vi "02_get_load_save.vi"() -> ()   [LabVIEW 2025]
uses:
  d34d51db-824d-4699-8c31-a07e0fcb91a3.vi
panel:
  out "NOTIFY_UI_Main_Switch_Buttons":T1
  out "var_New_Data":bool
types:
  T1 = cluster{"button_serial_connect":bool, "button_auto_sweep":bool, "button_tcp_connect":bool}
  T2 = cluster{"button_load_sxp":bool, "button_load_csv":bool, "button_save_s1p":bool, "button_save_s2p":bool, "button_single_sweep":bool, "tcp_load_cal":bool}
  T3 = cluster{"s11_data_available":bool, "s21_data_available":bool}
  T4 = cluster{"s11_available":bool, "s21_available":bool}
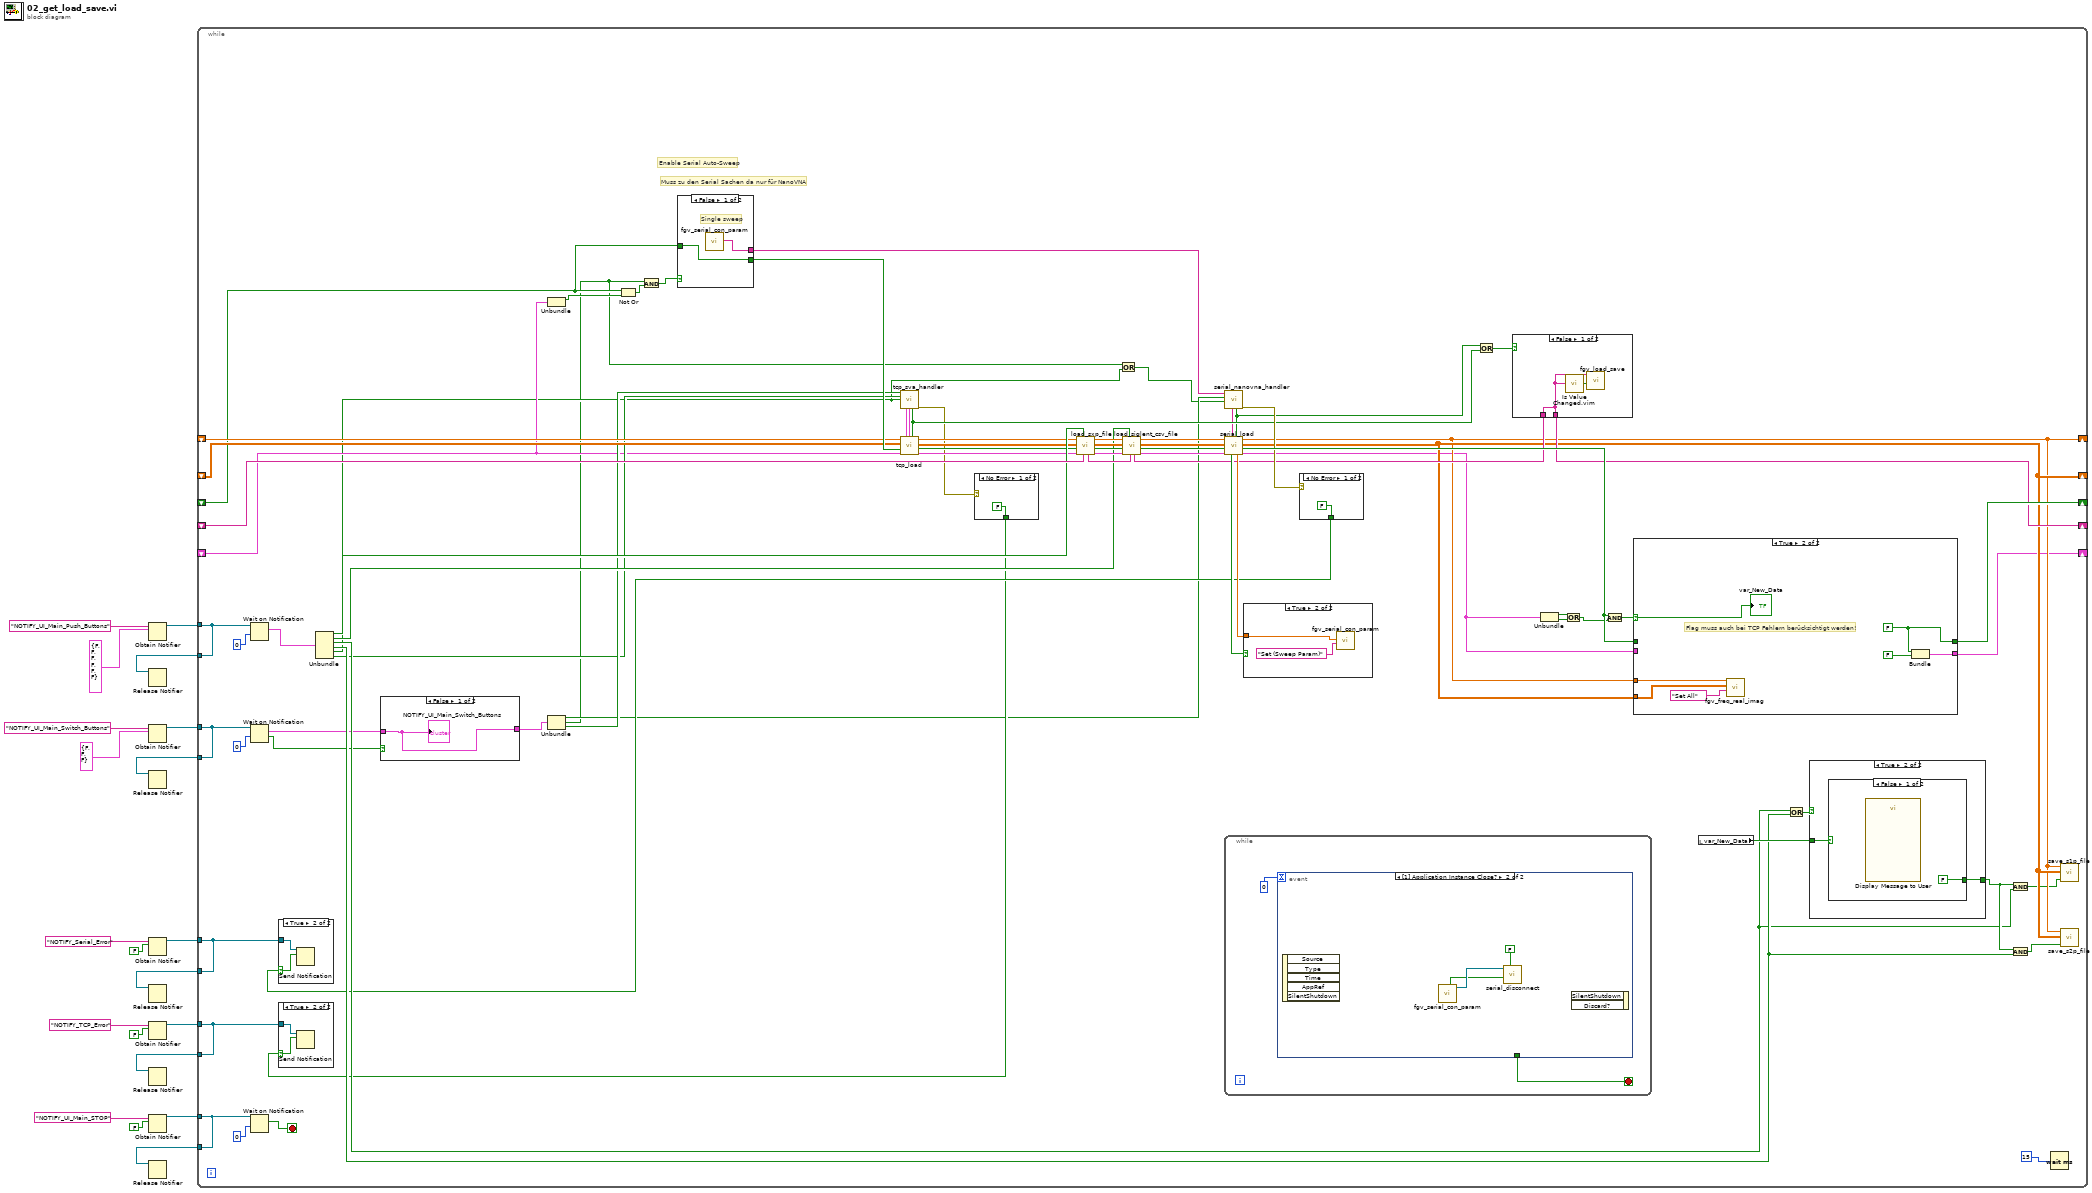
[diagram p0: block diagram]
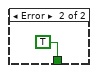
[diagram p2: hidden frame]
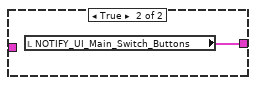
[diagram p4: hidden frame]
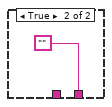
[diagram p6: hidden frame]
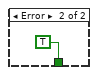
[diagram p7: hidden frame]
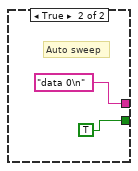
[diagram p8: hidden frame]
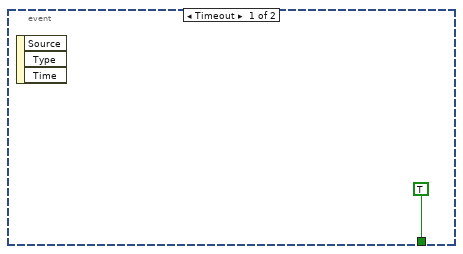
[diagram p10: hidden frame]
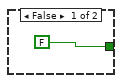
[diagram p11: hidden frame]
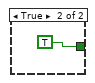
[diagram p12: hidden frame]
diagram:
  n1 = Obtain Notifier(name (unnamed)="NOTIFY_UI_Main_Push_Buttons", notification data type=T2 {"button_load_sxp"=FALSE, "button_load_csv"=FALSE, "button_save_s1p"=FALSE, "button_save_s2p"=FALSE, "button_single_sweep"=FALSE, "tcp_load_cal"=FALSE} ("output cluster")) -> (notifier out=w18:refnum<notifier>)  [unwired: 2 in, 2 out]
  n2 = Obtain Notifier(name (unnamed)="NOTIFY_UI_Main_Switch_Buttons", notification data type=T1 {"button_serial_connect"=FALSE, "button_auto_sweep"=FALSE, "button_tcp_connect"=FALSE} ("output cluster")) -> (notifier out=w9:refnum<notifier>)  [unwired: 2 in, 2 out]
  n3 = Obtain Notifier(name (unnamed)="NOTIFY_Serial_Error", notification data type=FALSE) -> (notifier out=w13:refnum<notifier>)  [unwired: 2 in, 2 out]
  n4 = Obtain Notifier(name (unnamed)="NOTIFY_TCP_Error", notification data type=FALSE) -> (notifier out=w1:refnum<notifier>)  [unwired: 2 in, 2 out]
  n5 = Obtain Notifier(name (unnamed)="NOTIFY_UI_Main_STOP", notification data type=FALSE) -> (notifier out=w14:refnum<notifier>)  [unwired: 2 in, 2 out]
  n6 = while {
    shift-right: [w95] -> _
    shift-left: _ -> [w24]
    shift-right: [w69] -> _
    shift-left: _ -> [w72]
    shift-right: [w70] -> _
    shift-left: _ -> [w73]
    shift-right: [w75] -> _
    shift-left: _ -> [w78]
    shift-right: [w63] -> _
    shift-left: _ -> [w28]
    tunnel: w18 -> [w57]
    tunnel: [w57] -> w19
    tunnel: w14 -> [w55]
    tunnel: [w55] -> w17
    tunnel: w13 -> [w48]
    tunnel: [w48] -> w10
    tunnel: w9 -> [w46]
    tunnel: [w46] -> w8
    tunnel: w1 -> [w37]
    tunnel: [w37] -> w4
    stop <- w53 stop-if-true
    # "Muss zu den Serial Sachen da nur für NanoVNA"
    # "Enable Serial Auto-Sweep"
    n7 = Wait on Notification(notifier=w57, timeout in ms (-1)=0) -> (notification=w56:T2)  [unwired: 2 in, 3 out]
    n8 = Wait on Notification(notifier=w46, timeout in ms (-1)=0) -> (notification=w43:T1, timed out?=w44:bool)  [unwired: 2 in, 2 out]
    n9 = Wait on Notification(notifier=w55, timeout in ms (-1)=0) -> (notification=w53:bool)  [unwired: 2 in, 3 out]
    n10 = Unbundle(w56) -> ("button_load_sxp"=w52:bool, "button_load_csv"=w51:bool, "button_save_s1p"=w49:bool, "button_save_s2p"=w50:bool, "button_single_sweep"=w23:bool, "tcp_load_cal"=w29:bool)
    n11 = case shown="False" w44 {
      tunnel: w43 -> [w101 _]
      tunnel: [w101 w102] -> w42
      frame False {
        "NOTIFY_UI_Main_Switch_Buttons" <- w101
      }
      frame True {
        n12 = local read "NOTIFY_UI_Main_Switch_Buttons"() -> (w102:T1)
      }
    }
    n13 = Unbundle(w28) -> ("s11_available"=w30:bool)  [unwired: 1 out]
    n14 = Unbundle(w42) -> ("button_serial_connect"=w25:bool, "button_auto_sweep"=w21:bool, "button_tcp_connect"=w35:bool)
    n15 = Not Or(1:w30, 2:w24) -> (0:w82:bool)
    n16 = And(x=w21, y=w82) -> (x .and. y?=w84:bool)
    n17 = case shown="False" w84 {
      tunnel: [w110 "data 0\n"] -> w81
      tunnel: [w111 TRUE ("new_freq_available")] -> w74
      tunnel: w24 -> [w111 _]
      frame False {
        # "Single sweep"
        n18 = call "fgv_serial_con_param.vi"() -> ("scan_command_get"=w110:string)  [unwired: 7 in, 4 out]
      }
      frame True {
        # "Auto sweep"
      }
    }
    n19 = call "tcp_sva_handler.vi"("button_tcp_connect"=w35, "button_tcp_load_cal"=w29, "button_get_trace_data"=w23) -> ("freq_range"=w34:cluster{"data out":string, "data out":string}, "data_out"=w33:cluster{"data out":string, "data out":string}, "new_data_available"=w32:bool, "error out"=w31:errorcluster)  [unwired: 9 in]
    n20 = call "tcp_load.vi"("freq_array_in"=w72, "freq_range"=w34, "data_in"=w33, "new_data_available"=w32, "data_array_in"=w73, "freq_available_in"=w74, "data_available_in"=w28) -> ("freq_array_out"=w41:dbl[], "data_array_out"=w40:dbl[][], "freq_available_out"=w39:bool, "data_available_out"=w38:T3)  [unwired: 5 in]
    n21 = case shown="No Error" w31 {
      tunnel: [FALSE TRUE] -> w36
      frame No Error {
      }
      frame Error {
      }
    }
    n22 = case shown="True" w36 {
      selector: w36 -> [_ w99]
      tunnel: w37 -> [_ w100]
      frame False {
      }
      frame True {
        n23 = Send Notification(notification=w99, notifier=w100) -> ()  [unwired: 1 in, 2 out]
      }
    }
    n24 = call "load_sxp_file.vi"("filename_in"=w78, "button_load_s1p"=w52, "data_available_in"=w38, "freq_available in"=w39, "data_array_in"=w40, "freq_array_in"=w41) -> ("data_available_out"=w91:T3, "freq_available out"=w92:bool, "data_array_out"=w93:dbl[][], "freq_array_out"=w94:dbl[], "filename_out"=w77:string)  [unwired: 1 in]
    n25 = Or(x=w21, y=w23) -> (x .or. y?=w22:bool)
    n26 = call "load_siglent_csv_file.vi"("filename_in"=w77, "button_load_csv"=w51, "data_available_in"=w91, "freq_available in"=w92, "s11_data_array_in"=w93, "freq_array_in"=w94) -> ("data_available_out"=w87:T3, "freq_available_out"=w88:bool, "s11_data_array_out"=w89:dbl[][], "freq_array_out"=w90:dbl[], "filename_out"=w76:string)  [unwired: 1 in]
    n27 = call "serial_nanovna_handler.vi"("button_get_trace_data"=w22, "button_serial_connect"=w25, "scan_command_get"=w81) -> ("error out"=w80:errorcluster, "new_data_available"=w26:bool, "read_buffer_out"=w27:string)  [unwired: 6 in]
    n28 = call "serial_load.vi"("new_data_available"=w26, "read_buffer_in"=w27, "data_available_in"=w87, "freq_available_in"=w88, "s11_data_array_in"=w89, "freq_array_in"=w90) -> ("data_available_out"=w62:T3, "freq_available_out"=w83:bool, "data_array_out"=w70:dbl[][], "freq_array_out"=w69:dbl[], "sweep_data"=w79:dbl[], "sweep_data_available"=w85:bool)
    n29 = while {
      stop <- w116 stop-if-true
      n30 = event shown="[1] Application Instance Close?" {
        selector: _ -> [_ _]
        dyn-events: _ -> [_ _]
        timeout: 0 -> [_ _]
        tunnel: [TRUE _] -> w116
        event Timeout {
          n31 = event-data() -> ()  [unwired: 1 in, 3 out]
        }
        event Application Instance Close? {
          n32 = event-data() -> ()  [unwired: 1 in, 5 out]
          n33 = call "fgv_serial_con_param.vi"() -> ("serial_port_get"=w120:refnum<visa-resource-name>, "serial_conn_get"=w119:bool)  [unwired: 7 in, 3 out]
          n34 = call "serial_disconnect.vi"("serial_disconnect"=FALSE, "serial_connected in"=w119, "VISA Refnum in"=w120) -> ()  [unwired: 7 in, 2 out]
          n35 = event-data() -> ()  [unwired: 3 in, 1 out]
        }
      }
    }
    n36 = case shown="True" w85 {
      tunnel: w79 -> [_ w114]
      frame False {
      }
      frame True {
        n37 = call "fgv_serial_con_param.vi"("mode"="Set (Sweep Param)", "sweep_param_set"=w114) -> ()  [unwired: 5 in, 5 out]
      }
    }
    n38 = case shown="No Error" w80 {
      tunnel: [FALSE TRUE] -> w47
      frame No Error {
      }
      frame Error {
      }
    }
    n39 = case shown="True" w47 {
      selector: w47 -> [_ w103]
      tunnel: w48 -> [_ w104]
      frame False {
      }
      frame True {
        n40 = Send Notification(notification=w103, notifier=w104) -> ()  [unwired: 1 in, 2 out]
      }
    }
    n41 = Or(x=w26, y=w32) -> (x .or. y?=w71:bool)
    n42 = case shown="False" w71 {
      tunnel: w76 -> [w105 _]
      tunnel: [w105 ""] -> w75
      frame False {
        n43 = call "Is Value Changed.vim"("value"=w105) -> ("changed or first call?"=w106:bool)
        n44 = call "fgv_load_save.vi"("write"=w106, "filename_set"=w105) -> ()  [unwired: 8 in, 2 out]
      }
      frame True {
      }
    }
    n45 = Unbundle(w62) -> ("s11_data_available"=w61:bool, "s21_data_available"=w60:bool)
    n46 = Or(x=w61, y=w60) -> (x .or. y?=w59:bool)
    n47 = And(x=w83, y=w59) -> (x .and. y?=w96:bool)
    n48 = case shown="True" w96 {
      selector: w96 -> [_ w130]
      tunnel: w69 -> [_ w133]
      tunnel: w70 -> [_ w132]
      tunnel: [w128 w134] -> w95
      tunnel: w83 -> [w128 _]
      tunnel: [w127 w135] -> w63
      tunnel: w62 -> [w127 _]
      frame False {
      }
      frame True {
        w134 = FALSE ("s11_available")
        # "Flag muss auch bei TCP Fehlern berücksichtigt werden!"
        n49 = call "fgv_freq_real_imag.vi"("mode"="Set All", "data_array_set"=w132, "freq_array_set"=w133) -> ()  [unwired: 5 in, 4 out]
        n50 = Bundle("s11_available"=w134, "s21_available"=FALSE) -> (w135:T4)  [unwired: 1 in]
        "var_New_Data" <- w130
      }
    }
    n51 = local read "var_New_Data"() -> (w68:bool)
    n52 = Or(x=w49, y=w50) -> (x .or. y?=w66:bool)
    n53 = case shown="True" w66 {
      tunnel: [FALSE w124] -> w64
      tunnel: w68 -> [_ w123]
      frame False {
      }
      frame True {
        n54 = case shown="False" w123 {
          tunnel: [FALSE TRUE] -> w124
          frame False {
            n55 = call "Display Message to User"() -> ()  [unwired: 10 in, 2 out]
          }
          frame True {
          }
        }
      }
    }
    n56 = And(x=w64, y=w49) -> (x .and. y?=w67:bool)
    n57 = And(x=w64, y=w50) -> (x .and. y?=w65:bool)
    n58 = Wait (ms)(milliseconds to wait=u32 15) -> ()  [unwired: 1 out]
    n59 = call "save_s1p_file.vi"("button_save_s1p"=w67, "data_array_in"=w70, "freq_array_in"=w69) -> ()  [unwired: 9 in]
    n60 = call "save_s2p_file.vi"("button_save_s2p"=w65, "data_array_in"=w70, "freq_array_in"=w69) -> ()  [unwired: 9 in]
  }
  n61 = Release Notifier(notifier=w19) -> ()  [unwired: 2 in, 3 out]
  n62 = Release Notifier(notifier=w8) -> ()  [unwired: 2 in, 3 out]
  n63 = Release Notifier(notifier=w10) -> ()  [unwired: 2 in, 3 out]
  n64 = Release Notifier(notifier=w4) -> ()  [unwired: 2 in, 3 out]
  n65 = Release Notifier(notifier=w17) -> ()  [unwired: 2 in, 3 out]
